vi "Disconnect.vi"(8 "error in (no error)":errorcluster, 11 "PLCHandler in":refnum<class "PLCHandler.lvclass">) -> (0 "error out":errorcluster, 3 "PLCHandler out":refnum<class "PLCHandler.lvclass">)   [LabVIEW 2022 SP3, in "PLCHandler.lvlib" / "PLCHandler.lvclass"]
uses:
  PLCHandler.lvclass
  PLCHandler.lvclass/PLCHandler.ctl
  <vilib>/NI/Modbus Library/API/Master/Modbus Master.lvclass
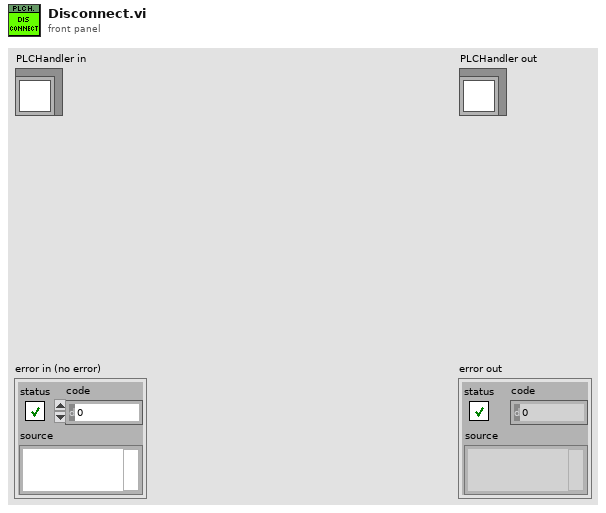
[diagram p1: front panel]
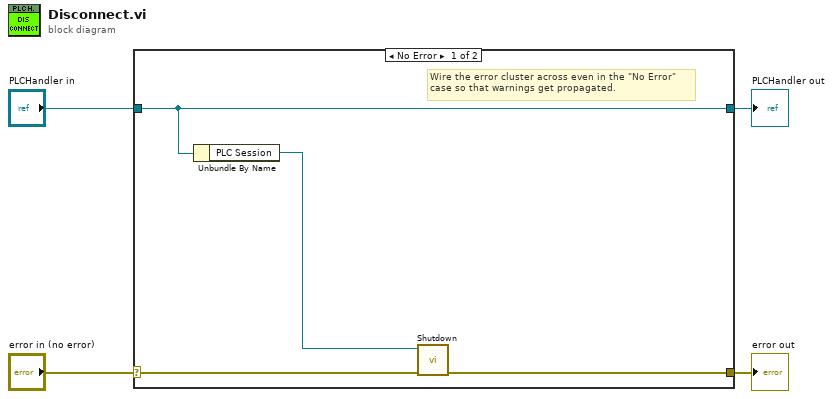
[diagram p0: block diagram]
diagram:
  n1 = case shown="No Error" "error in (no error)" {
    selector: "error in (no error)" -> [w8 w10]
    tunnel: [w6 w10] -> w3
    tunnel: [w7 w9] -> w1
    tunnel: "PLCHandler in" -> [w7 w9]
    frame No Error {
      # "Wire the error cluster across even in the \"No Error\"\ncase so that warnings get propagated."
      n2 = Unbundle By Name(w7) -> ("PLC Session"=w5:refnum<class "Modbus Master.lvclass">)
      n3 = call-dynamic "Shutdown.vi"("error in"=w8, "Modbus master in"=w5) -> ("error out"=w6:errorcluster)  [unwired: 9 in]
    }
    frame Error {
    }
  }
  "error out" <- w3
  "PLCHandler out" <- w1
